vi "Handle Command.vi"(8 "error in (no error)":errorcluster, 9 "Data":variant, 10 "Command":string, 11 "Inst.Magneto in":refnum<class "Inst.Magneto.lvclass">) -> (0 "error out":errorcluster, 1 "Processed Data":variant, 2 "Command":string, 3 "Inst.Magneto out":refnum<class "Inst.Magneto.lvclass">)   [LabVIEW 2019, in "Inst.Magneto.lvclass"]
uses:
  Inst.Magneto.lvclass
  Typedefs/Inst.Magneto.Commands--Enum.ctl
  Inst.Magneto.lvclass/Inst.Magneto.ctl
  Typedefs/Inst.Magneto.getAll--Cluster.ctl
  9aec49fd-fe04-463a-be35-b7075f22e824.vi
  9aec49fd-fe04-463a-be35-b7075f22e824.vi/144aaf49-b203-4cd0-b857-13a99ed5042e.vi
  9aec49fd-fe04-463a-be35-b7075f22e824.vi/971e7276-0b9c-479d-bfbf-39c63a00d2c0.vi
  <vilib>/Utility/Data Type/Get Type Information.vi
  <vilib>/JDP Science/JSONtext/JSON text to Variant.vi
  <vilib>/JDP Science/JSONtext/LVClass Serializer/JSONtext LVClass Serializer.lvclass
  <userlib>/LevyLab/Instrument Framework/Instrument Types/VSource/Instrument.VSource.lvclass
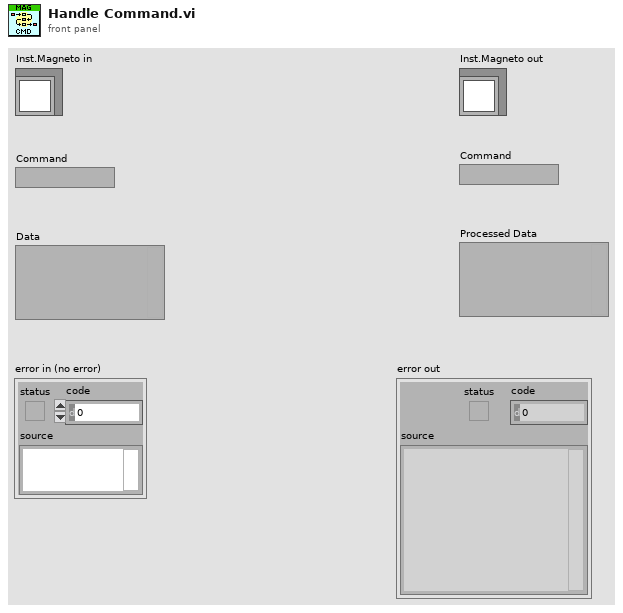
[diagram p1: front panel]
types:
  T1 = typedef "Inst.Magneto.lvclass/Inst.Magneto.Commands--Enum.ctl" = enum16{"GetRead", "Read", "Clear Values"}
  T2 = typedef "Inst.Magneto.lvclass/Inst.Magneto.getAll--Cluster.ctl" = cluster{"AllString":string}
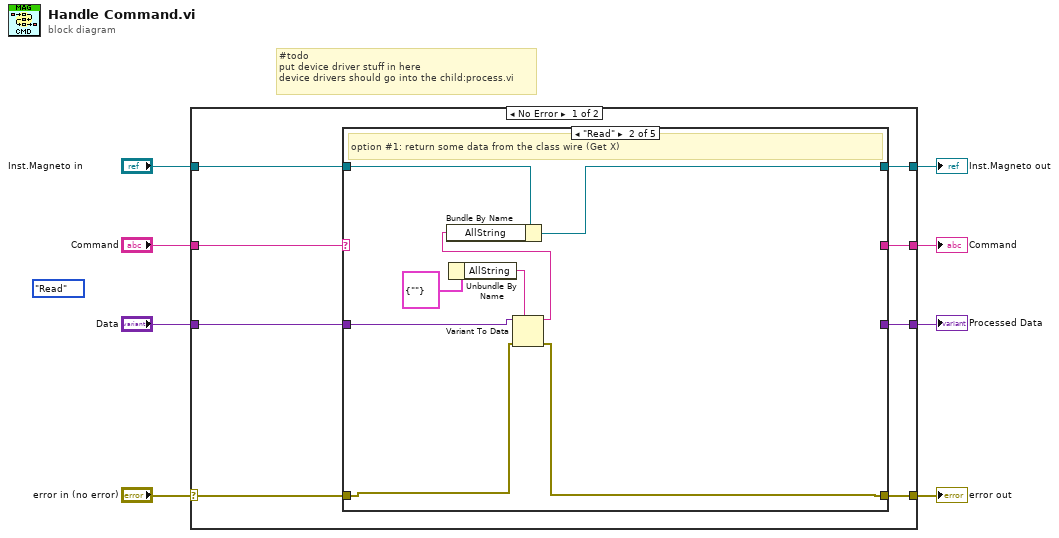
[diagram p0: block diagram]
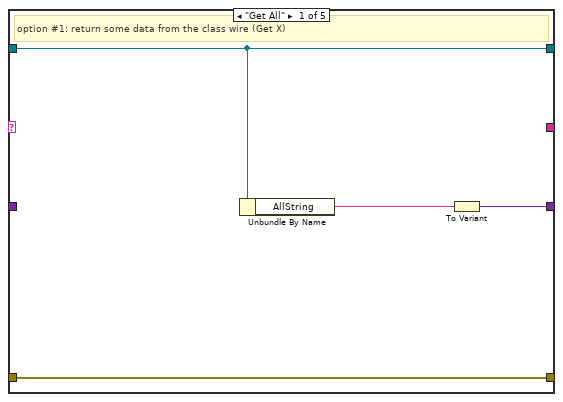
[diagram p2: hidden frame]
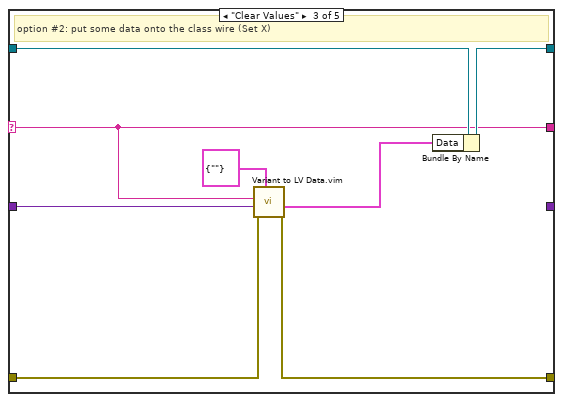
[diagram p3: hidden frame]
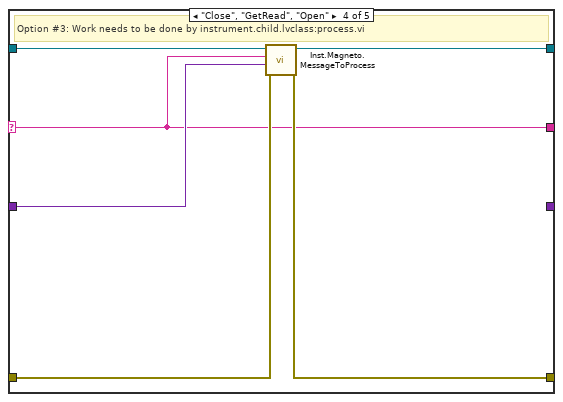
[diagram p4: hidden frame]
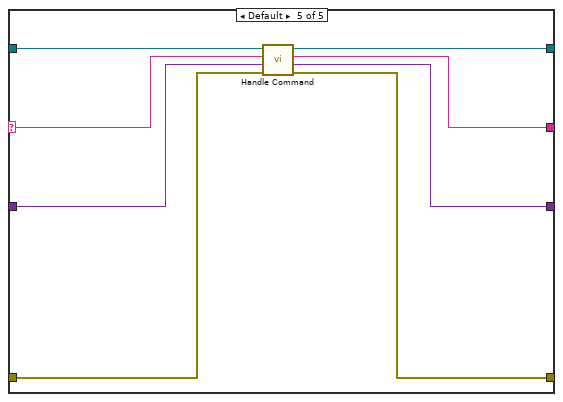
[diagram p5: hidden frame]
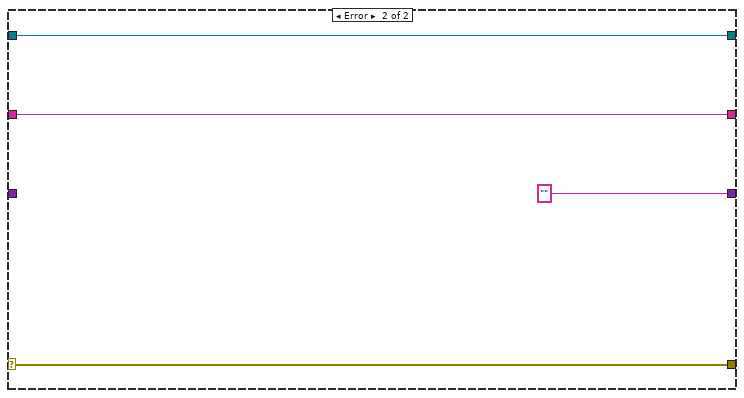
[diagram p6: hidden frame]
diagram:
  (unwired) Inst.Magneto.Commands--Enum."Read" ("Commands")
  # "#todo\nput device driver stuff in here\ndevice drivers should go into the child:process.vi"
  n1 = case shown="No Error" "error in (no error)" {
    selector: "error in (no error)" -> [w10 w54]
    tunnel: [w12 w54] -> w6
    tunnel: [w14 w53] -> w5
    tunnel: "Inst.Magneto in" -> [w15 w53]
    tunnel: "Command" -> [w16 w51]
    tunnel: [w13 "" ("String")] -> w3
    tunnel: "Data" -> [w9 _]
    tunnel: [w11 w51] -> w1
    frame No Error {
      n2 = case shown="\"Read\"" w16 {
        selector: w16 -> [_ _ w30 w37 w44]
        tunnel: w15 -> [w19 w27 w36 w42 w48]
        tunnel: [w19 w28 w35 w41 w45] -> w14
        tunnel: [w17 _ _ _ w47] -> w13
        tunnel: w10 -> [w18 w26 w34 w40 w49]
        tunnel: w9 -> [_ w24 w32 w38 w50]
        tunnel: [w18 w25 w33 w39 w46] -> w12
        tunnel: [_ _ w30 w37 w43] -> w11
        frame "Get All" {
          # "option #1: return some data from the class wire (Get X)"
          n3 = Unbundle By Name(w19) -> ("AllString"=w20:string)
          n4 = To Variant(anything=w20) -> (Variant=w17:variant)
        }
        frame "Read" {
          # "option #1: return some data from the class wire (Get X)"
          n5 = Unbundle By Name(T2 {"AllString"=""} ("getAll")) -> ("AllString"=w21:string)
          n6 = Variant To Data(error in=w26, type=w21, Variant=w24) -> (data=w23:string, error out=w25:errorcluster)
          n7 = Bundle By Name(cluster=w27, "AllString"=w23) -> (w28:refnum<class "Inst.Magneto.lvclass">)
        }
        frame "Clear Values" {
          # "option #2: put some data onto the class wire (Set X)"
          n8 = call "Variant to LV Data.vim"("type"=T2 {"AllString"=""} ("getAll"), "error in (no error)"=w34, "JSON Data in"=w32, "Command"=w30) -> ("error out"=w33:errorcluster, "Data out"=w31:T2)  [unwired: 4 in, 2 out]
          n9 = Bundle By Name(cluster=w36, "Data"=w31) -> (w35:refnum<class "Inst.Magneto.lvclass">)
        }
        frame "Close", "GetRead", "Open" {
          # "Option #3: Work needs to be done by instrument.child.lvclass:process.vi"
          n10 = call "Inst.Magneto.MessageToProcess.vi"("error in (no error)"=w40, "Data"=w38, "Command"=w37, "Inst.Magneto in"=w42) -> ("error out"=w39:errorcluster, "Inst.Magneto out"=w41:refnum<class "Inst.Magneto.lvclass">)  [unwired: 6 in]
        }
        frame Default {
          n11 = call-parent "Handle Command.vi"("error in (no error)"=w49, "Data"=w50, "Command"=w44, "Instrument in"=w48) -> ("error out"=w46:errorcluster, "Processed Data"=w47:variant, "Command"=w43:string, "Instrument out"=w45:refnum<class "Inst.Magneto.lvclass">)  [unwired: 4 in]
        }
      }
    }
    frame Error {
    }
  }
  "error out" <- w6
  "Inst.Magneto out" <- w5
  "Command" <- w1
  "Processed Data" <- w3
